vi "Write Sync Box Setup.vi"(8 "error in (no error)":errorcluster, 9 "Remote Port":u32=2000, 10 "Address":string="192.168.254.183", 11 "Interface in":refnum<class "Interface.lvclass">) -> (0 "error out":errorcluster, 3 "Interface out":refnum<class "Interface.lvclass">)   [LabVIEW 2018, in "Interface.lvclass"]
uses:
  Interface.lvclass
  Interface.lvclass/Interface.ctl
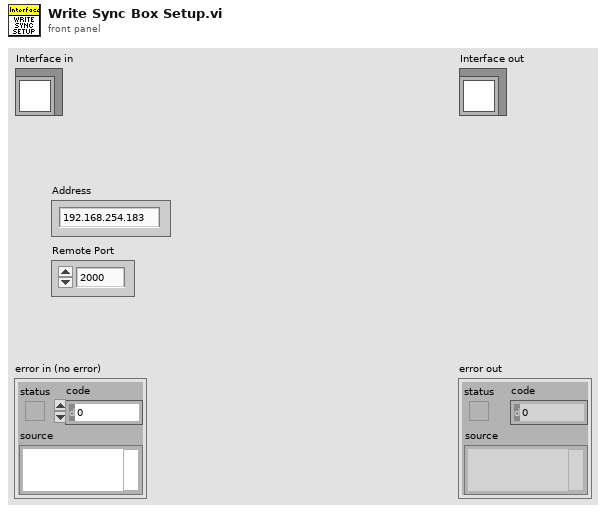
[diagram p1: front panel]
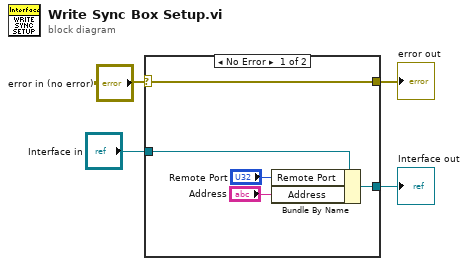
[diagram p0: block diagram]
diagram:
  n1 = case shown="No Error" "error in (no error)" {
    selector: "error in (no error)" -> [w9 w11]
    tunnel: [w9 w11] -> w3
    tunnel: [w5 w10] -> w1
    tunnel: "Interface in" -> [w8 w10]
    frame No Error {
      n2 = Bundle By Name(cluster=w8, "Remote Port"="Remote Port", "Address"="Address") -> (w5:refnum<class "Interface.lvclass">)
    }
    frame Error {
    }
  }
  "error out" <- w3
  "Interface out" <- w1
